vi "add.vi"() -> ()   [LabVIEW 2021]
panel:
  out "x+y":dbl
  in  "y":dbl
  in  "x":dbl
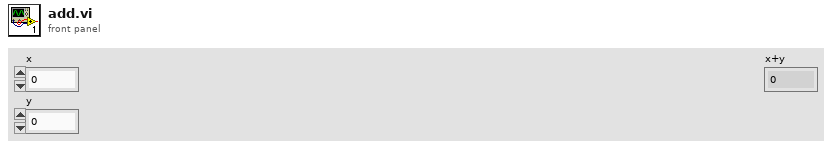
[diagram p1: front panel]
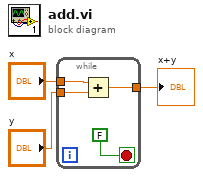
[diagram p0: block diagram]
diagram:
  n1 = while {
    tunnel: "x" -> [w7]
    tunnel: "y" -> [w6]
    tunnel: [w5] -> w1
    stop <- FALSE stop-if-true
    n2 = Add(x=w7, y=w6) -> (x+y=w5:dbl)
  }
  "x+y" <- w1
